vi "SECoP_dataGetType.vi"(8 "error in (no error)":errorcluster, 10 "SECoP_dataPtr":T1 {"ptr64" format="%.0x"; "ptr32" format="%.0x"}, 11 "DLL path (in)":T2) -> (0 "error out":errorcluster, 2 "data type description":string, 3 "DLL path (out)":T2)   [LabVIEW 2023, in "SECoP.lvlib"]
doc: "Call <b>\"SECoP_dataGetType.vi\"</b> to return the data type description of this value. See SECoP protocol definition.\n\n<b>DLL path</b> input and output of cluster from \"SECoP-Initialize.vi\"\n<b>SECoP_dataPtr</b> created data\n<b>data type description</b> SECoP data type description"
uses:
  SECoP.lvlib
  SECoP-libraries.ctl
  SECoP-data.ctl
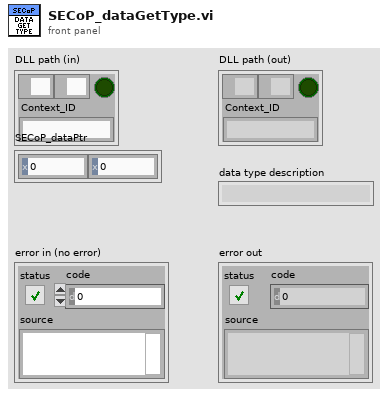
[diagram p1: front panel]
types:
  T1 = typedef "SECoP.lvlib/SECoP-data.ctl" = cluster{"ptr32":u32, "ptr64":u64}
  T2 = typedef "SECoP.lvlib/SECoP-libraries.ctl" = cluster{"serverDLL":path, "variantDLL":path, "cleanup_mode":bool, "Context_ID":string}
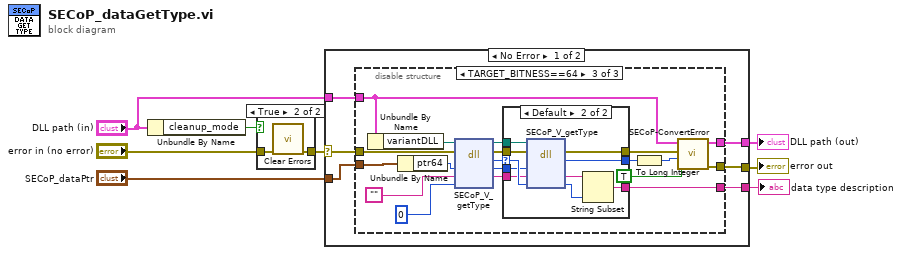
[diagram p0: block diagram]
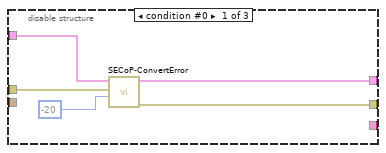
[diagram p3: hidden frame]
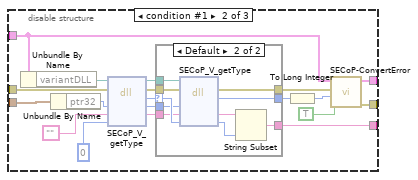
[diagram p4: hidden frame]
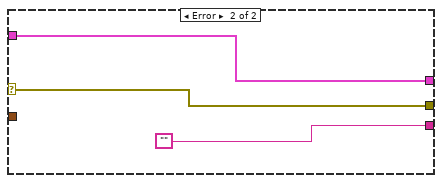
[diagram p7: hidden frame]
diagram:
  n1 = Unbundle By Name("DLL path (in)") -> ("cleanup_mode"=w6:bool)
  n2 = case shown="True" w6 {
    tunnel: "error in (no error)" -> [w9 w11]
    tunnel: [w9 w10] -> w4
    frame False {
    }
    frame True {
      n3 = call <vilib>:"Clear Errors.vi"("error in (no error)"=w11) -> ("error out"=w10:errorcluster)  [unwired: 5 in, 1 out]
    }
  }
  n4 = case shown="No Error" w4 {
    selector: w4 -> [w17 w88]
    tunnel: "DLL path (in)" -> [w12 w89]
    tunnel: [w14 w89] -> w8
    tunnel: [w15 w88] -> w7
    tunnel: [w16 ""] -> w3
    tunnel: "SECoP_dataPtr" -> [w13 _]
    frame No Error {
      n5 = disable-structure shown="TARGET_BITNESS==64" {
        disable-tunnel: w17 -> [w19 w41 w73]
        disable-tunnel: [_ w32 w64] -> w16
        disable-tunnel: [w21 w26 w58] -> w15
        disable-tunnel: [w22 w27 w59] -> w14
        disable-tunnel: w13 -> [_ w39 w71]
        disable-tunnel: w12 -> [w20 w23 w55]
        frame condition #0 {
          n6 = call "SECoP-ConvertError.vi"("return code"=-20, "error in (no error)"=w19, "DLL path (in)"=w20) -> ("error out"=w21:errorcluster, "DLL path (out)"=w22:T2)  [unwired: 7 in]
        }
        frame condition #1 {
          n7 = Unbundle By Name(w23) -> ("variantDLL"=w24:path)
          n8 = Unbundle By Name(w39) -> ("ptr32"=w38:u32)
          n9 = dll-call lib="Z:/Praktische_Aufgaben/SECoP-LabVIEW2015/32bit/SECoP32.dll" fn="SECoP_V_getType"(path in=w24, error in=w41, "pData"=w38, "szBuffer"="", "iBufferSize"=u32 0 ("BufferSize")) -> (path out=w35:path, error out=w34:errorcluster, "return type"=w36:u32, "pData"=w25:u32, "szBuffer"=w33:string)  [unwired: 2 in]
          n10 = case shown="Default" w36 {
            selector: w36 -> [w43 w51]
            tunnel: w35 -> [_ w54]
            tunnel: w34 -> [w44 w53]
            tunnel: [w44 w52] -> w28
            tunnel: [w43 w50] -> w29
            tunnel: w33 -> [w42 w49]
            tunnel: [w42 w46] -> w32
            tunnel: w25 -> [_ w45]
            frame 0 {
            }
            frame Default {
              n11 = dll-call lib="Z:/Praktische_Aufgaben/SECoP-LabVIEW2015/32bit/SECoP32.dll" fn="SECoP_V_getType"(path in=w54, error in=w53, "pData"=w45, "szBuffer"=w49, "iBufferSize"=w51) -> (error out=w52:errorcluster, "return type"=w50:u32, "szBuffer"=w48:string, "iBufferSize"=w47:u32)  [unwired: 2 in, 1 out]
              n12 = String Subset(string=w48, length (rest)=w47) -> (substring=w46:string)  [unwired: 1 in]
            }
          }
          n13 = To Long Integer(number=w29) -> (32bit integer=w30:i32)
          n14 = call "SECoP-ConvertError.vi"("return is boolean"=TRUE, "return code"=w30, "error in (no error)"=w28, "DLL path (in)"=w23) -> ("error out"=w26:errorcluster, "DLL path (out)"=w27:T2)  [unwired: 6 in]
        }
        frame condition #2 (active) {
          n15 = Unbundle By Name(w55) -> ("variantDLL"=w56:path)
          n16 = Unbundle By Name(w71) -> ("ptr64"=w70:u64)
          n17 = dll-call lib="Z:/Praktische_Aufgaben/SECoP-LabVIEW2015/32bit/SECoP32.dll" fn="SECoP_V_getType"(path in=w56, error in=w73, "pData"=w70, "szBuffer"="", "iBufferSize"=u32 0 ("BufferSize")) -> (path out=w67:path, error out=w66:errorcluster, "return type"=w68:u32, "pData"=w57:u64, "szBuffer"=w65:string)  [unwired: 2 in]
          n18 = case shown="Default" w68 {
            selector: w68 -> [w75 w83]
            tunnel: w67 -> [_ w86]
            tunnel: w66 -> [w76 w85]
            tunnel: [w76 w84] -> w60
            tunnel: [w75 w82] -> w61
            tunnel: w65 -> [w74 w81]
            tunnel: [w74 w78] -> w64
            tunnel: w57 -> [_ w77]
            frame 0 {
            }
            frame Default {
              n19 = dll-call lib="Z:/Praktische_Aufgaben/SECoP-LabVIEW2015/32bit/SECoP32.dll" fn="SECoP_V_getType"(path in=w86, error in=w85, "pData"=w77, "szBuffer"=w81, "iBufferSize"=w83) -> (error out=w84:errorcluster, "return type"=w82:u32, "szBuffer"=w80:string, "iBufferSize"=w79:u32)  [unwired: 2 in, 1 out]
              n20 = String Subset(string=w80, length (rest)=w79) -> (substring=w78:string)  [unwired: 1 in]
            }
          }
          n21 = To Long Integer(number=w61) -> (32bit integer=w62:i32)
          n22 = call "SECoP-ConvertError.vi"("return is boolean"=TRUE, "return code"=w62, "error in (no error)"=w60, "DLL path (in)"=w55) -> ("error out"=w58:errorcluster, "DLL path (out)"=w59:T2)  [unwired: 6 in]
        }
      }
    }
    frame Error {
    }
  }
  "DLL path (out)" <- w8
  "error out" <- w7
  "data type description" <- w3
